vi "WPL_close waveform.vi"(8 "error in (no error)":errorcluster, 9 "Variant":variant, 10 "Command":T1, 11 "WPL Comm in":refnum<class "WPL Comm.lvclass">) -> (0 "error out":errorcluster)   [LabVIEW 2020, in "Internal Comm Classes.lvlib" / "WPL Comm.lvclass"]
uses:
  WPL Comm.lvclass
  WPL Command.ctl
  WPL Comm.lvclass/WPL Comm.ctl
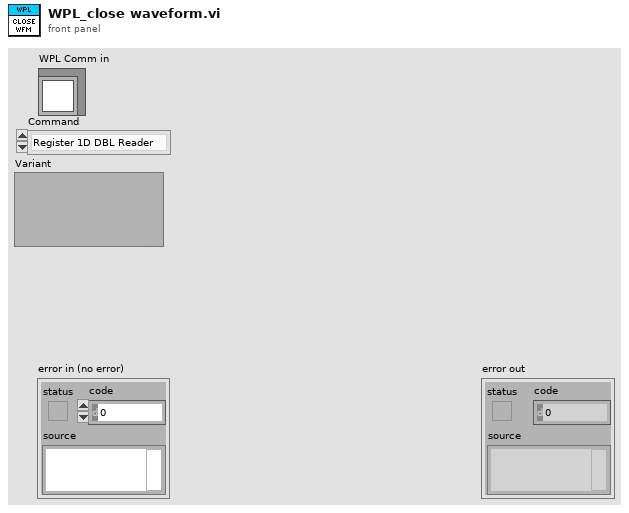
[diagram p1: front panel]
types:
  T1 = typedef "Internal Comm Classes.lvlib/WPL Comm.lvclass/WPL Command.ctl" = enum16{"Register 1D DBL Reader", "Unregister 1D DBL Reader", "Register 1D DBL Writer", "Register 2D DBL Writer", "Unregister 1D DBL Writer", "Unregister 2D DBL Writer", "DBL WFM Start", "WFM 1D DBL Data", "WFM 2D DBL Data", "Shut down", "Handle Error", "Register 1D CDB Reader", "Unregister 1D CDB Reader", "Register 1D CDB Writer", "Unregister 1D CDB Writer", "Register 2D CDB Writer", "Unregister 2D CDB Writer", "WFM 1D CDB Data", "WFM 2D CDB Data", "CDB WFM Start", "Error Shutdown", "Register Streams", "Unregister Streams", "Delete All Streams", "Get WFM DTs", "DBL WFM Multi Start", "CDB WFM Multi Start"}
  T2 = typedef "Internal Comm Classes.lvlib/WPL Comm.lvclass/WPL Command Queue ref.ctl" = refnum<queue>
  T3 = typedef "Internal Comm Classes.lvlib/WPL Comm.lvclass/Waveform error queue.ctl" = refnum<queue>
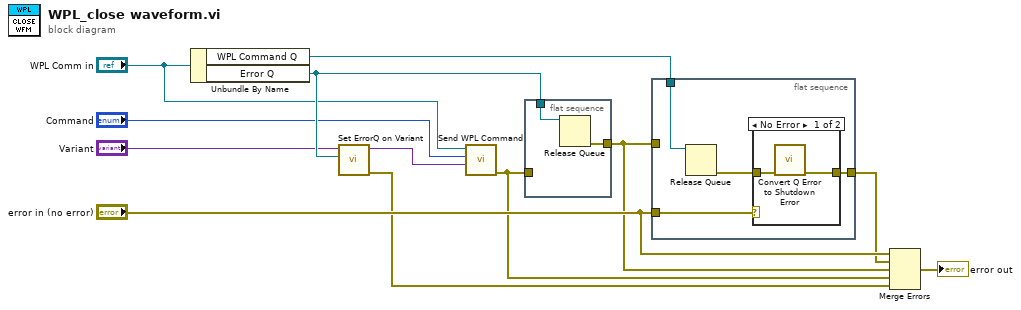
[diagram p0: block diagram]
diagram:
  n1 = Unbundle By Name("WPL Comm in") -> ("WPL Command Q"=w11:T2, "Error Q"=w12:T3)
  n2 = call "Set ErrorQ on Variant.vi"("Queue in"=w12, "Variant in"="Variant") -> ("error out"=w2:errorcluster, "Variant out"=w7:variant)  [unwired: 7 in, 1 out]
  n3 = call "Send WPL Command.vi"("Variant"=w7, "Command"="Command", "WPL Comm"="WPL Comm in") -> ("error out"=w3:errorcluster)  [unwired: 7 in, 1 out]
  n4 = flat-sequence {
    tunnel: w12 -> [w14]
    tunnel: w3 -> [_]
    tunnel: [w13] -> w4
    frame #0 {
      n5 = Release Queue(queue=w14) -> (error out=w13:errorcluster)  [unwired: 2 in, 2 out]
    }
  }
  n6 = flat-sequence {
    tunnel: w11 -> [w18]
    tunnel: w4 -> [_]
    tunnel: "error in (no error)" -> [w17]
    tunnel: [w15] -> w5
    frame #0 {
      n7 = Release Queue(queue=w18) -> (error out=w16:errorcluster)  [unwired: 2 in, 2 out]
      n8 = case shown="No Error" w17 {
        tunnel: w16 -> [w20 w21]
        tunnel: [w19 w21] -> w15
        frame No Error {
          n9 = call "Convert Q Error to Shutdown Error.vi"("error in (no error)"=w20) -> ("error out"=w19:errorcluster)  [unwired: 10 in]
        }
        frame Error {
        }
      }
    }
  }
  n10 = Merge Errors("error in (no error)", w5, w4, w3, w2) -> (→"error out":errorcluster)
